vi "Disabled.vi"(7 "Robot Mode":T2, 10 "Match Info":T1={"Autonomous Elapsed Seconds"=0.0, "TeleOp Elapsed Seconds"=0.0, "Disabled Elapsed Seconds"=0.0, "Visited Autonomous"=FALSE, "Visited TeleOp"=FALSE, "Visited Disabled"=FALSE, "Autonomous Settings"={"Autonomous Style"=enum."Independent", "VI Refnum"=refnum}}, 11 "Call Context":T3) -> ()   [LabVIEW 2020]
doc: "This VI is called each time a disabled packet is received from the DS. It is often used to prepare for the next robot mode, to calibrate sensors, etc."
uses:
  <vilib>/Rock Robotics/WPI/DriverStation/WPI_DriverStationDerivedRobotMode.ctl
  <vilib>/Rock Robotics/WPI/DriverStation/WPI_DriverStationRobotMode2.ctl
  <vilib>/Rock Robotics/WPI/DriverStation/WPI_DriverStationMatch Info.ctl
  <vilib>/Rock Robotics/WPI/Joystick/XBox Buttons Indexer.ctl
  <vilib>/Rock Robotics/WPI/Utilities/WPI_GetSetVariantRefNum.vi
  Robot Global Data.vi
  <vilib>/Rock Robotics/WPI/ThirdParty/Phoenix-LabVIEW/CANCoder/Get/CTRE_Phoenix_CANcoder_GetSensorData.vi
  <vilib>/Rock Robotics/Network Tables/NT Write Number.vi
  <vilib>/Rock Robotics/Network Tables/NT Write String.vi
  <vilib>/Rock Robotics/Network Tables/NT Write Boolean.vi
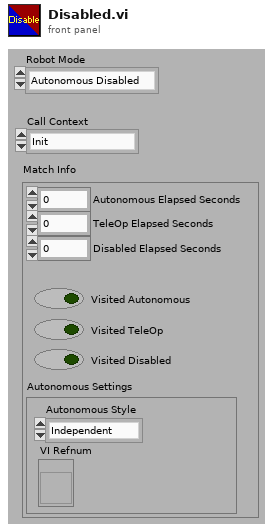
[diagram p1: front panel]
types:
  T1 = typedef "WPI_DriverStationMatch Info.ctl" = cluster{"Autonomous Elapsed Seconds":dbl, "TeleOp Elapsed Seconds":dbl, "Disabled Elapsed Seconds":dbl, "Visited Autonomous":bool, "Visited TeleOp":bool, "Visited Disabled":bool, "Autonomous Settings":cluster{"Autonomous Style":enum16{"Iterative", "Independent"}, "VI Refnum":refnum<vi>}}
  T2 = typedef "WPI_DriverStationRobotMode2.ctl" = enum16{"Autonomous Disabled", "Autonomous Enabled", "Teleop Disabled", "Teleop Enabled", "Disconnected", "Finish", "Test Disabled", "Test Enabled", "Emergency Stopped"}
  T3 = typedef "WPI_DriverStationDerivedRobotMode.ctl" = enum16{"Init", "Execute", "Stop"}
  T4 = typedef "XBox Buttons Indexer.ctl" = enum16{"A", "B", "X", "Y", "Left Bumper", "Right Bumper", "Back", "Start", "Left Joystick", "Right Joystick"}
  T5 = typedef "Absolute Angle TypeDef.ctl" = cluster{"leftFrontAbsoluteAngle":dbl, "leftRearAbsoluteAngle":dbl, "rightFrontAbsoluteAngle":dbl, "rightRearAbsoluteAngle":dbl}
  T6 = typedef "WPI_JoystickDevRef.ctl" = cluster{"Device":T7}
  T7 = typedef "WPI_JoystickDeviceEnum.ctl" = enum16{"USB 0", "USB 1", "USB 2", "USB 3", "USB 4", "USB 5"}
  T8 = typedef "WPI_DriverStationAllianceInfo.ctl" = enum16{"Red", "Blue", "Invalid"}
  T9 = typedef "CTRE_Phoenix_CANcoder_DeviceRef.ctl" = cluster{"DeviceStatus":errorcluster, "Device Number":u8, "Handle":u64, "UsageFrame":u32, "Library Path":path}
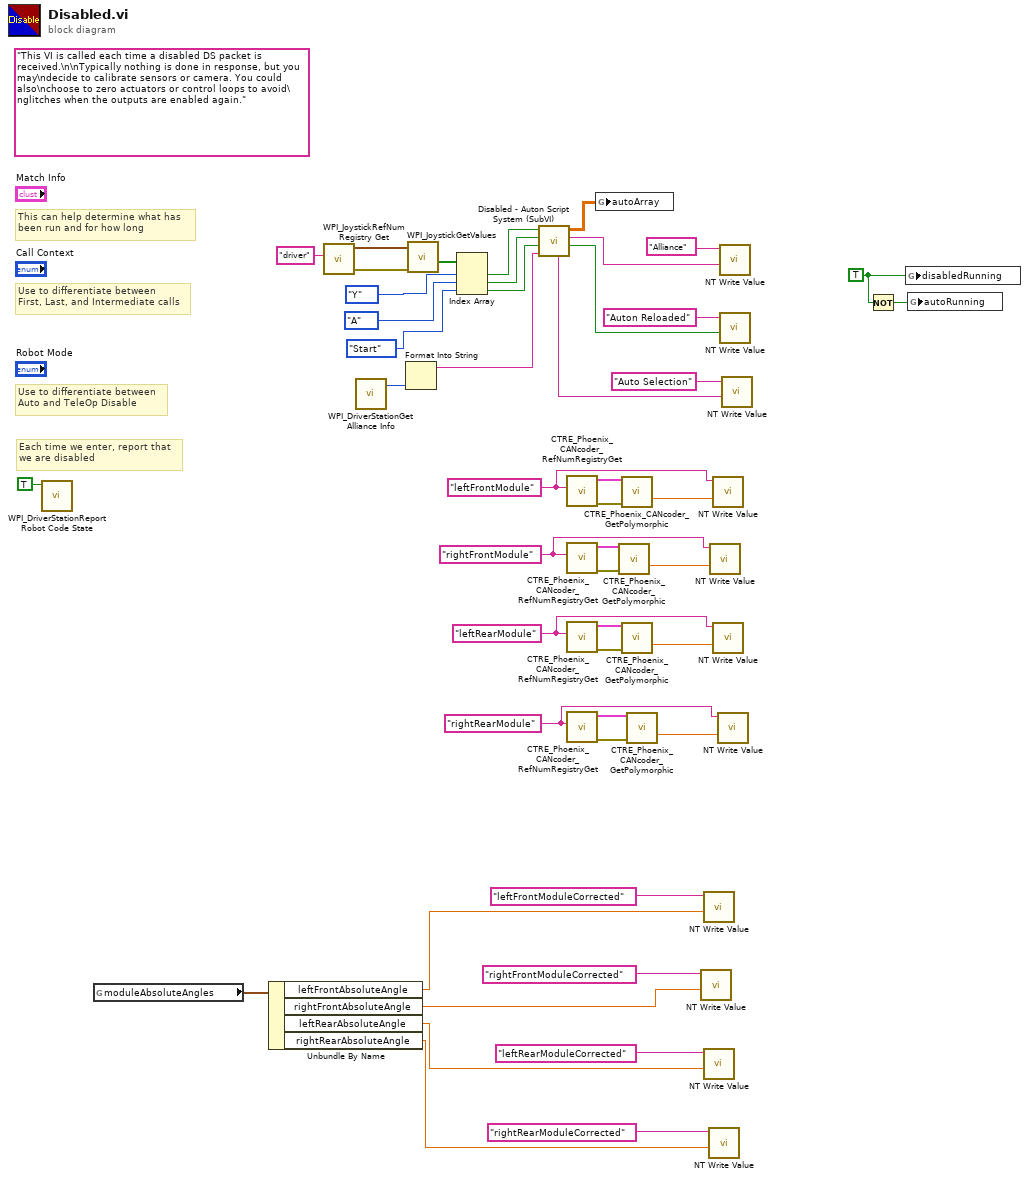
[diagram p0: block diagram]
diagram:
  w10 = "rightRearModule" ("refnum name")
  w14 = "leftRearModule" ("refnum name")
  w18 = "rightFrontModule" ("refnum name")
  w22 = "leftFrontModule" ("refnum name")
  w30 = TRUE ("Enable Vision")
  (unwired) "This VI is called each time a disabled DS packet is received.\n\nTypically nothing is done in response, but you may\ndecide to calibrate sensors or camera. You could also\nchoose to zero actuators or control loops to avoid\nglitches when the outputs are enabled again."
  # "Each time we enter, report that\nwe are disabled"
  # "Use to differentiate between\nFirst, Last, and Intermediate calls"
  # "This can help determine what has\nbeen run and for how long"
  # "Use to differentiate between\nAuto and TeleOp Disable"
  n1 = call <vilib>:"WPI_DriverStationReport Robot Code State.vi"("Disabled"=TRUE ("Autonomous")) -> ()  [unwired: 10 in, 1 out]
  n2 = global read "Robot Global Data.vi" "moduleAbsoluteAngles"() -> (w5:T5)
  n3 = Unbundle By Name(w5) -> ("leftFrontAbsoluteAngle"=w4:dbl, "rightFrontAbsoluteAngle"=w3:dbl, "leftRearAbsoluteAngle"=w2:dbl, "rightRearAbsoluteAngle"=w1:dbl)
  n4 = call <vilib>:"WPI_JoystickRefNum Registry Get.vi"("refnum name"="driver") -> ("error out"=w44:errorcluster, "JoystickDevRef"=w45:T6)  [unwired: 9 in]
  n5 = call <vilib>:"WPI_DriverStationGet Alliance Info.vi"() -> ("Alliance"=w32:T8)  [unwired: 6 in, 5 out]
  n6 = Format Into String(w32) -> (resulting string=w31:string)  [unwired: 3 in, 1 out]
  n7 = call <vilib>:"WPI_JoystickGetValues.vi"("error in (no error)"=w44, "JoystickDevRef"=w45) -> ("Buttons"=w43:bool[])  [unwired: 5 in, 4 out]
  n8 = Index Array(array=w43, index #1=XBox_Buttons_Indexer."Y" ("XBox Buttons"), index #2=XBox_Buttons_Indexer."A" ("XBox Buttons"), index #3=XBox_Buttons_Indexer."Start" ("XBox Buttons")) -> (element #1=w42:bool, element #2=w41:bool, element #3=w40:bool)
  n9 = call "Disabled - Auton Script System (SubVI).vi"("Alliance Color Input"=w31, "Reload File Names"=w40, "Down File"=w41, "Up File"=w42) -> ("Files Reloaded"=w35:bool, "Alliance Color"=w36:string, "all rows"=w33:dbl[][], "File Name"=w34:string)  [unwired: 2 in, 2 out]
  n10 = call <vilib>:"CTRE_Phoenix_CANcoder_RefNumRegistryGet.vi"("refnum name"=w22) -> ("error out"=w24:errorcluster, "CTRE_CANcoder_DeviceRef"=w25:T9)  [unwired: 9 in]
  n11 = call <vilib>:"CTRE_Phoenix_CANcoder_RefNumRegistryGet.vi"("refnum name"=w18) -> ("error out"=w20:errorcluster, "CTRE_CANcoder_DeviceRef"=w21:T9)  [unwired: 9 in]
  n12 = call <vilib>:"CTRE_Phoenix_CANcoder_RefNumRegistryGet.vi"("refnum name"=w14) -> ("error out"=w16:errorcluster, "CTRE_CANcoder_DeviceRef"=w17:T9)  [unwired: 9 in]
  n13 = call <vilib>:"CTRE_Phoenix_CANcoder_RefNumRegistryGet.vi"("refnum name"=w10) -> ("error out"=w12:errorcluster, "CTRE_CANcoder_DeviceRef"=w13:T9)  [unwired: 9 in]
  n14 = global write "Robot Global Data.vi" "autoArray"(w33) -> ()
  n15 = call-poly <vilib>:"CTRE_Phoenix_CANcoder_GetPolymorphic.vi"("CTRE_CANcoder_DeviceRef"=w21, "error in"=w20) -> ("Absolute Position"=w19:dbl)  [unwired: 9 in, 4 out]
  n16 = call-poly <vilib>:"CTRE_Phoenix_CANcoder_GetPolymorphic.vi"("CTRE_CANcoder_DeviceRef"=w25, "error in"=w24) -> ("Absolute Position"=w23:dbl)  [unwired: 9 in, 4 out]
  n17 = call-poly <vilib>:"CTRE_Phoenix_CANcoder_GetPolymorphic.vi"("CTRE_CANcoder_DeviceRef"=w17, "error in"=w16) -> ("Absolute Position"=w15:dbl)  [unwired: 9 in, 4 out]
  n18 = call-poly <vilib>:"CTRE_Phoenix_CANcoder_GetPolymorphic.vi"("CTRE_CANcoder_DeviceRef"=w13, "error in"=w12) -> ("Absolute Position"=w11:dbl)  [unwired: 9 in, 4 out]
  n19 = call-poly <vilib>:"NT Write Value.vi"("Numeric"=w3, "Name"="rightFrontModuleCorrected" ("refnum name")) -> ()  [unwired: 9 in, 1 out]
  n20 = call-poly <vilib>:"NT Write Value.vi"("Numeric"=w4, "Name"="leftFrontModuleCorrected" ("refnum name")) -> ()  [unwired: 9 in, 1 out]
  n21 = call-poly <vilib>:"NT Write Value.vi"("Numeric"=w2, "Name"="leftRearModuleCorrected" ("refnum name")) -> ()  [unwired: 9 in, 1 out]
  n22 = call-poly <vilib>:"NT Write Value.vi"("Numeric"=w1, "Name"="rightRearModuleCorrected" ("refnum name")) -> ()  [unwired: 9 in, 1 out]
  n23 = call-poly <vilib>:"NT Write Value.vi"("Numeric"=w19, "Name"=w18) -> ()  [unwired: 9 in, 1 out]
  n24 = call-poly <vilib>:"NT Write Value.vi"("Numeric"=w23, "Name"=w22) -> ()  [unwired: 9 in, 1 out]
  n25 = call-poly <vilib>:"NT Write Value.vi"("Numeric"=w15, "Name"=w14) -> ()  [unwired: 9 in, 1 out]
  n26 = call-poly <vilib>:"NT Write Value.vi"("Numeric"=w11, "Name"=w10) -> ()  [unwired: 9 in, 1 out]
  n27 = call-poly <vilib>:"NT Write Value.vi"("String"=w36, "Name"="Alliance") -> ()  [unwired: 9 in, 1 out]
  n28 = call-poly <vilib>:"NT Write Value.vi"("Boolean"=w35, "Name"="Auton Reloaded") -> ()  [unwired: 9 in, 1 out]
  n29 = call-poly <vilib>:"NT Write Value.vi"("String"=w34, "Name"="Auto Selection") -> ()  [unwired: 9 in, 1 out]
  n30 = Not(x=w30) -> (.not. x?=w29:bool)
  n31 = global write "Robot Global Data.vi" "disabledRunning"(w30) -> ()
  n32 = global write "Robot Global Data.vi" "autoRunning"(w29) -> ()
